vi "Handle Error.vi"(8 "error in (no error)":errorcluster, 11 "GenNet Protocol in":refnum<class "GenNet Variant Protocol.lvclass">) -> (0 "error out":errorcluster, 1 "Add Info for Error Broadcast":string, 2 "Module ID for Error Broadcast":i32=-1, 3 "GenNet Protocol out":refnum<class "GenNet Variant Protocol.lvclass">)   [LabVIEW 2022 SP3, in "hse-gennet.lvlib" / "GenNet Variant Protocol.lvclass"]
doc: "____\nHAMPEL SOFTWARE ENGINEERING v3.8.0 (2023-12-18 14:41)"
uses:
  GenNet Variant Protocol.lvclass
  GenNet Protocol.lvclass
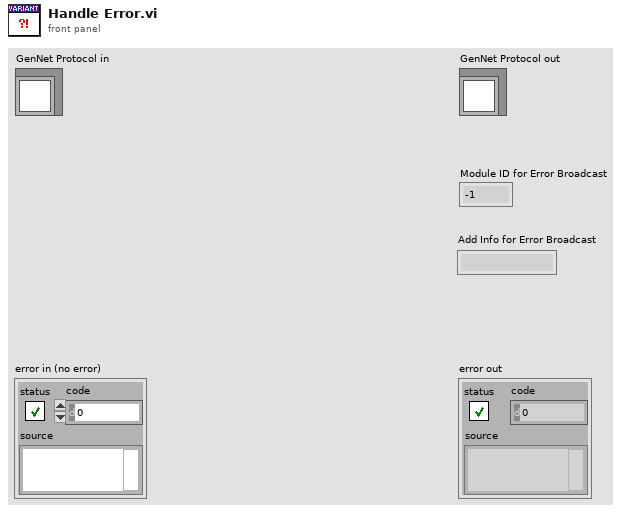
[diagram p1: front panel]
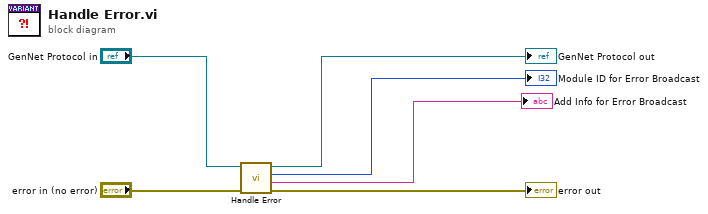
[diagram p0: block diagram]
diagram:
  n1 = call-parent "Handle Error.vi"("error in (no error)"="error in (no error)", "GenNet Protocol in"="GenNet Protocol in") -> ("error out"=→"error out":errorcluster, "Add Info for Error Broadcast"=→"Add Info for Error Broadcast":string, "Module ID for Error Broadcast"=→"Module ID for Error Broadcast":i32, "GenNet Protocol out"=→"GenNet Protocol out":refnum<class "GenNet Variant Protocol.lvclass">)  [unwired: 6 in]
